vi "XY Graph Save Plot.vi"(6 "Delimiter (TAB)":string="\t", 8 "Error In":errorcluster, 9 "Plot Index":i32, 11 "XYGraph Ref":T1) -> (0 "Error Out":errorcluster, 1 "File Path":path, 2 "Plot Name":string, 3 "XYGraph Ref":T1, 4 "Cancelled":bool, 5 "Graph Name":string)   [LabVIEW 2019, in "XY Graph Add-Ons.lvlib"]
uses:
  XY Graph Add-Ons.lvlib
  XY Graph Refnum.ctl
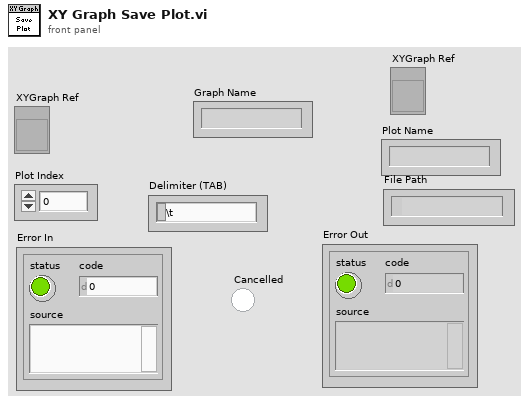
[diagram p1: front panel]
types:
  T1 = typedef "XY Graph Add-Ons.lvlib/XY Graph Refnum.ctl" = refnum<vi>
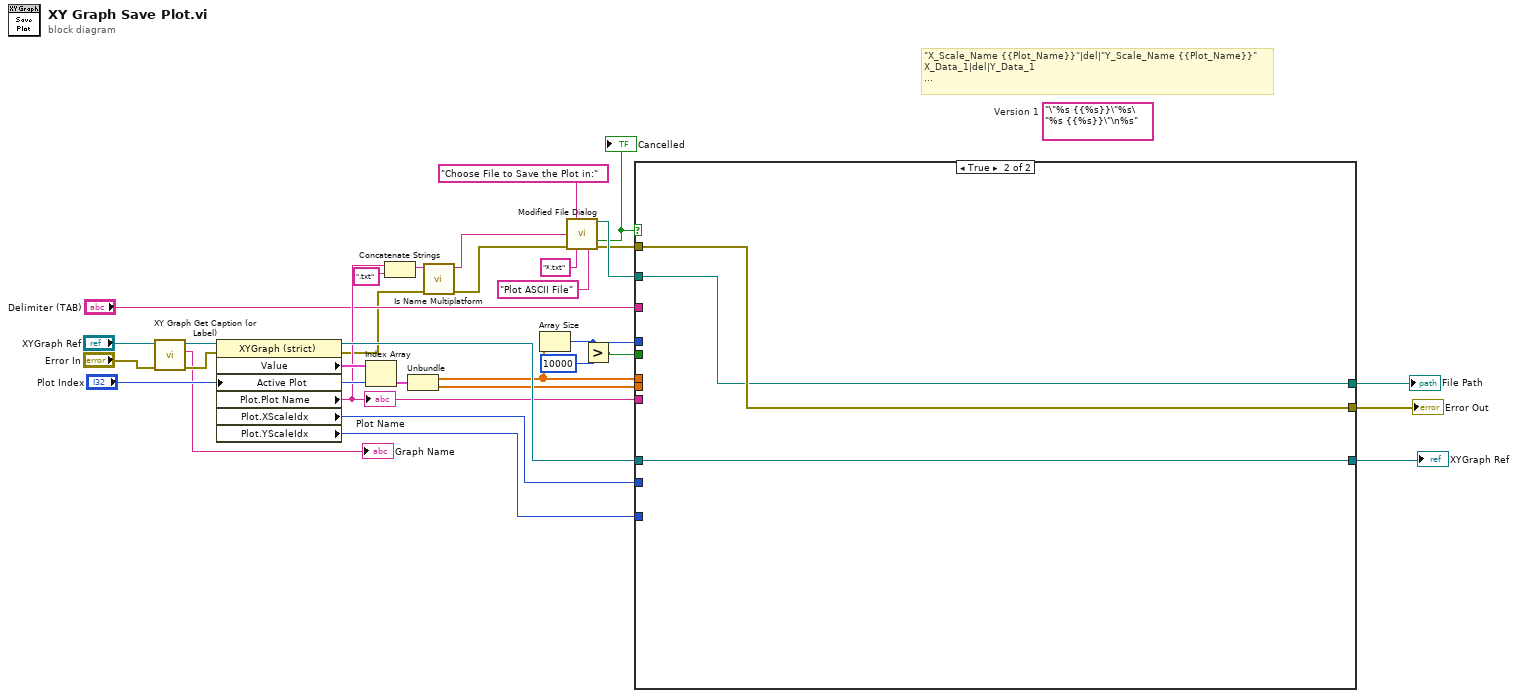
[diagram p0: block diagram]
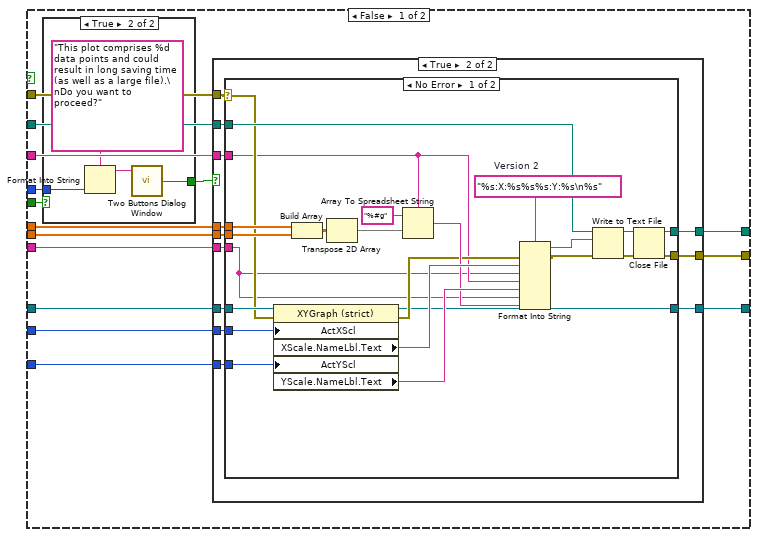
[diagram p2: hidden frame]
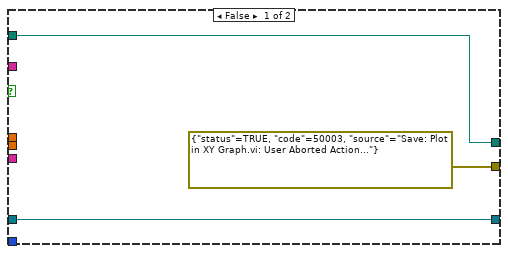
[diagram p3: hidden frame]
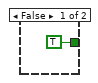
[diagram p5: hidden frame]
diagram:
  (unwired) "\"%s {{%s}}\"%s\"%s {{%s}}\"\n%s"  # Version 1
  # "\"X_Scale_Name {{Plot_Name}}\"|del|\"Y_Scale_Name {{Plot_Name}}\"\nX_Data_1|del|Y_Data_1\n..."
  n1 = call "XY Graph Get Caption (or Label).vi"("error in (no error)"="Error In", "XYGraph in"="XYGraph Ref") -> ("error out"=w6:errorcluster, "Caption (or Label) Text"=→"Graph Name":string, "XYGraph out"=w8:T1)  [unwired: 7 in]
  n2 = property class="XYGraph (strict)"(reference=w8, error in=w6, "Active Plot"="Plot Index") -> (reference out=w28:T1, error out=w10:errorcluster, "Value"=w31:cluster{"X Array":dbl[], "Y Array":dbl[]}[], "Plot.Plot Name"=w24:string, "Plot.XScaleIdx"=w27:u32, "Plot.YScaleIdx"=w26:u32)
  "Plot Name" <- w24
  n3 = Index Array(array=w31, index="Plot Index") -> (element=w29:cluster{"X Array":dbl[], "Y Array":dbl[]})
  n4 = Concatenate Strings(w24, ".txt" ("string")) -> (w17:string)
  n5 = Unbundle(w29) -> ("X Array"=w14:dbl[], "Y Array"=w25:dbl[])
  n6 = call <vilib>:"Is Name Multiplatform.vi"("error in (no error)"=w10, "filename"=w17) -> ("error out"=w16:errorcluster, "suggested filename"=w15:string)  [unwired: 5 in, 3 out]
  n7 = Array Size(array=w14) -> (size(s)=w12:i32)
  n8 = call "Modified File Dialog.vi"("prompt"="Choose File to Save the Plot in:", "suggested filename"=w15, "error in (no error)"=w16, "pattern"="*.txt" ("pattern (all files)"), "pattern label"="Plot ASCII File") -> ("selected path"=w23:path, "Cancelled"=w4:bool, "error out"=w20:errorcluster)  [unwired: 7 in, 1 out]
  "Cancelled" <- w4
  n9 = Greater?(x=w12, y=10000) -> (0:w11:bool)
  n10 = case shown="True" w4 {
    tunnel: w28 -> [w47 w96]
    tunnel: w27 -> [w46 _]
    tunnel: w26 -> [w45 _]
    tunnel: w25 -> [w44 _]
    tunnel: w24 -> [w43 _]
    tunnel: w23 -> [w42 w94]
    tunnel: [w41 w95] -> w22
    tunnel: [w40 w94] -> w21
    tunnel: w20 -> [w39 w95]
    tunnel: "Delimiter (TAB)" -> [w38 _]
    tunnel: w14 -> [w37 _]
    tunnel: w12 -> [w36 _]
    tunnel: w11 -> [w35 _]
    tunnel: [w33 w96] -> w9
    frame False {
      n11 = case shown="True" w35 {
        tunnel: w36 -> [_ w92]
        tunnel: [TRUE ("T button?") w90] -> w34
        frame False {
        }
        frame True {
          n12 = Format Into String(format string="This plot comprises %d data points and could result in long saving time (as well as a large file).\nDo you want to proceed?", w92) -> (resulting string=w91:string)  [unwired: 2 in, 1 out]
          n13 = call "Two Buttons Dialog Window.vi"("Message"=w91) -> ("OK?"=w90:bool)  [unwired: 2 in]
        }
      }
      n14 = case shown="True" w34 {
        tunnel: w47 -> [w48 w62]
        tunnel: w46 -> [_ w61]
        tunnel: w45 -> [_ w60]
        tunnel: w44 -> [_ w59]
        tunnel: w43 -> [_ w58]
        tunnel: w42 -> [w49 w57]
        tunnel: [errorcluster {"status"=TRUE, "code"=50003, "source"="Save: Plot in XY Graph.vi: User Aborted Action..."} ("error IO") w56] -> w41
        tunnel: [w49 w55] -> w40
        tunnel: w39 -> [_ w54]
        tunnel: w38 -> [_ w53]
        tunnel: w37 -> [_ w52]
        tunnel: [w48 w51] -> w33
        frame False {
        }
        frame True {
          n15 = case shown="No Error" w54 {
            selector: w54 -> [w68 w88]
            tunnel: w62 -> [w86 w87]
            tunnel: w61 -> [w85 _]
            tunnel: w60 -> [w84 _]
            tunnel: w52 -> [w83 _]
            tunnel: w59 -> [w82 _]
            tunnel: w58 -> [w65 _]
            tunnel: w57 -> [w72 _]
            tunnel: [w66 w88] -> w56
            tunnel: [w64 _] -> w55
            tunnel: w53 -> [w67 _]
            tunnel: [w63 w87] -> w51
            frame No Error {
              w78 = "%s:X:%s%s%s:Y:%s\n%s"  # Version 2
              n16 = property class="XYGraph (strict)"(reference=w86, error in=w68, "ActXScl"=w85, "ActYScl"=w84) -> (reference out=w63:T1, error out=w74:errorcluster, "XScale.NameLbl.Text"=w77:string, "YScale.NameLbl.Text"=w76:string)
              n17 = Build Array(w83, w82) -> (w81:dbl[][])
              n18 = Transpose 2D Array(2D array=w81) -> (transposed array=w80:dbl[][])
              n19 = Array To Spreadsheet String(delimiter (Tab)=w67, array=w80, 3:"%#g" ("format string")) -> (spreadsheet string=w75:string)
              n20 = Format Into String(format string=w78, error in=w74, w77, w65, w67, w76, w65, w75) -> (resulting string=w73:string, error out=w71:errorcluster)  [unwired: 1 in]
              n21 = Write to Text File(file (use dialog)=w72, text=w73, error in=w71) -> (refnum out=w70:refnum<file>, error out=w69:errorcluster)  [unwired: 1 in, 1 out]
              n22 = Close File(refnum=w70, error in=w69) -> (path=w64:path, error out=w66:errorcluster)
            }
            frame Error {
            }
          }
        }
      }
    }
    frame True {
    }
  }
  "Error Out" <- w22
  "File Path" <- w21
  "XYGraph Ref" <- w9
